vi "串口.vi"() -> ()   [LabVIEW 2012]
uses:
  <vilib>/Instr/_visa.llb/VISA Configure Serial Port (Instr).vi
  <vilib>/Utility/file.llb/Read From Spreadsheet File (I64).vi
  <vilib>/Utility/file.llb/Write To Spreadsheet File (I64).vi
panel:
  out "接收字节缓冲区":u8[](array[numeric])
  in  "选项卡控件":enum32{"帧采集", "采集信号", "信号回放"}(tab)
  out "时间：年月日-小时-分":string
  in  "保存数据格式":path=path "data.txt"
  out "卡车声":bool
  out "脚步声":bool
  in  "布尔 2":bool=TRUE
  in  "baud rate":u32=19200 caption="波特率"
  in  "VISA resource name":refnum<visa-resource-name>="COM1" caption="串口号"
  out "bytes read":u32=7 caption="读取的字节"
  in  "write":bool caption="写入"
  in  "string to write":string="*IDN?\n" caption="写入字符串"
  in  "read":bool=TRUE caption="读取"
  in  "data bits":u16=8 caption="数据比特" min=5 max=8 step=1
  in  "parity":u16(ring) caption="奇偶" items=["无", "奇", "偶", "标记", "空格"]
  in  "stop bits":u16(ring)=10 caption="停止位" items=["1.0"=10, "1.5"=15, "2.0"=20]
  in  "flow control":u16(ring) caption="流程控制" items=["无"=0, "XON/XOFF"=1, "RTS/CTS"=2, "DTR/DSR"=4]
  in  "delay before read (ms)":u32=1 caption="读取前延时(ms)"
  out "波形显示":cluster{u32, u32}(graph)
  out "read string":string="*IDN?\n" caption="读取字符串"
  in  "布尔":bool
  in  "保存帧格式":path=path "frame.txt"
  out "波形显示 2":u32[](graph) caption="波形显示"
  in  "数据位数":u16(ring)=8 items=["8"=8, "16"=16, "32"=32]
  in  "信号回放按键":bool
  out "波形显示 3":i64[][](graph) caption="波形显示"
  in  "数据格式文件":path=path "data.txt"
  # "1. 帧格式：\n    0xAA 类型 数据低字位 数据高字节 保留字节 保留字节 异或校验字节\n2. 类型： 0: nothing 1: 声方向 2: 目标类型 3: 过零率\n3. 此处无浏览按钮的路径都使用当前VI的相对路径"
  # "注：数据先低字节后高字节"
  # "1. 回放的信号文件必须是数据格式存储的文件\n2. 此处使用绝对路径"
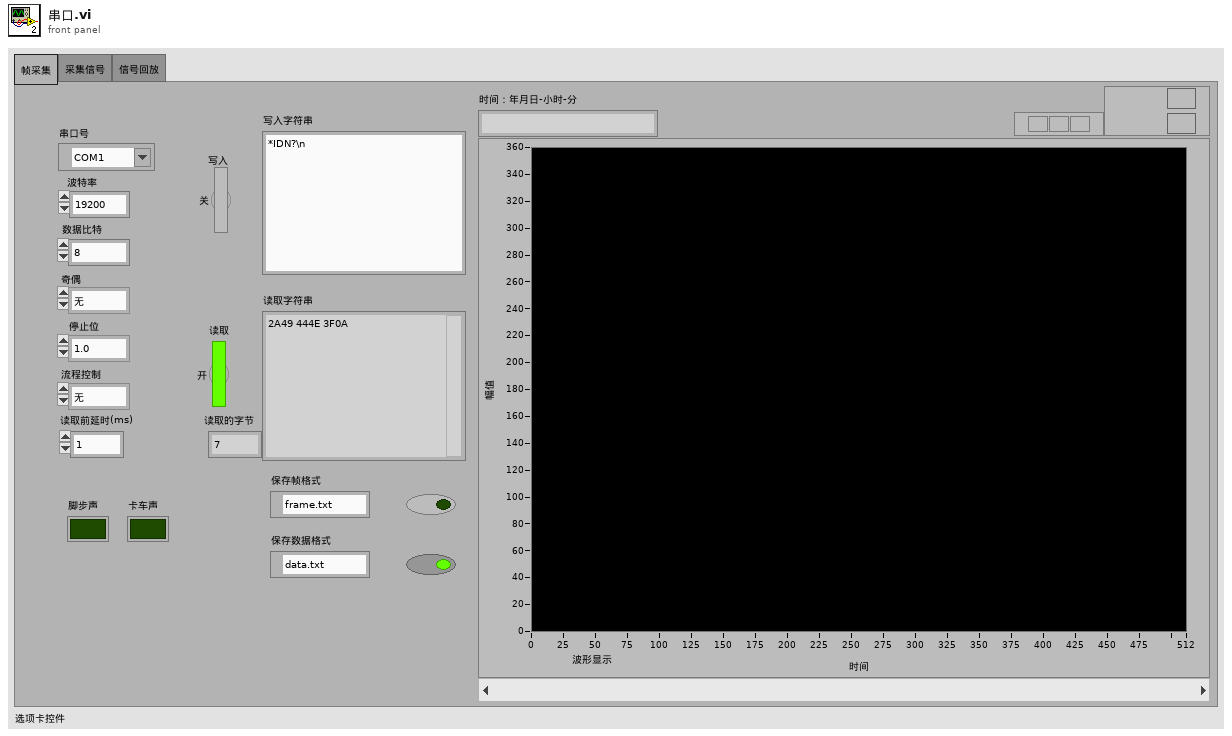
[diagram p1: front panel]
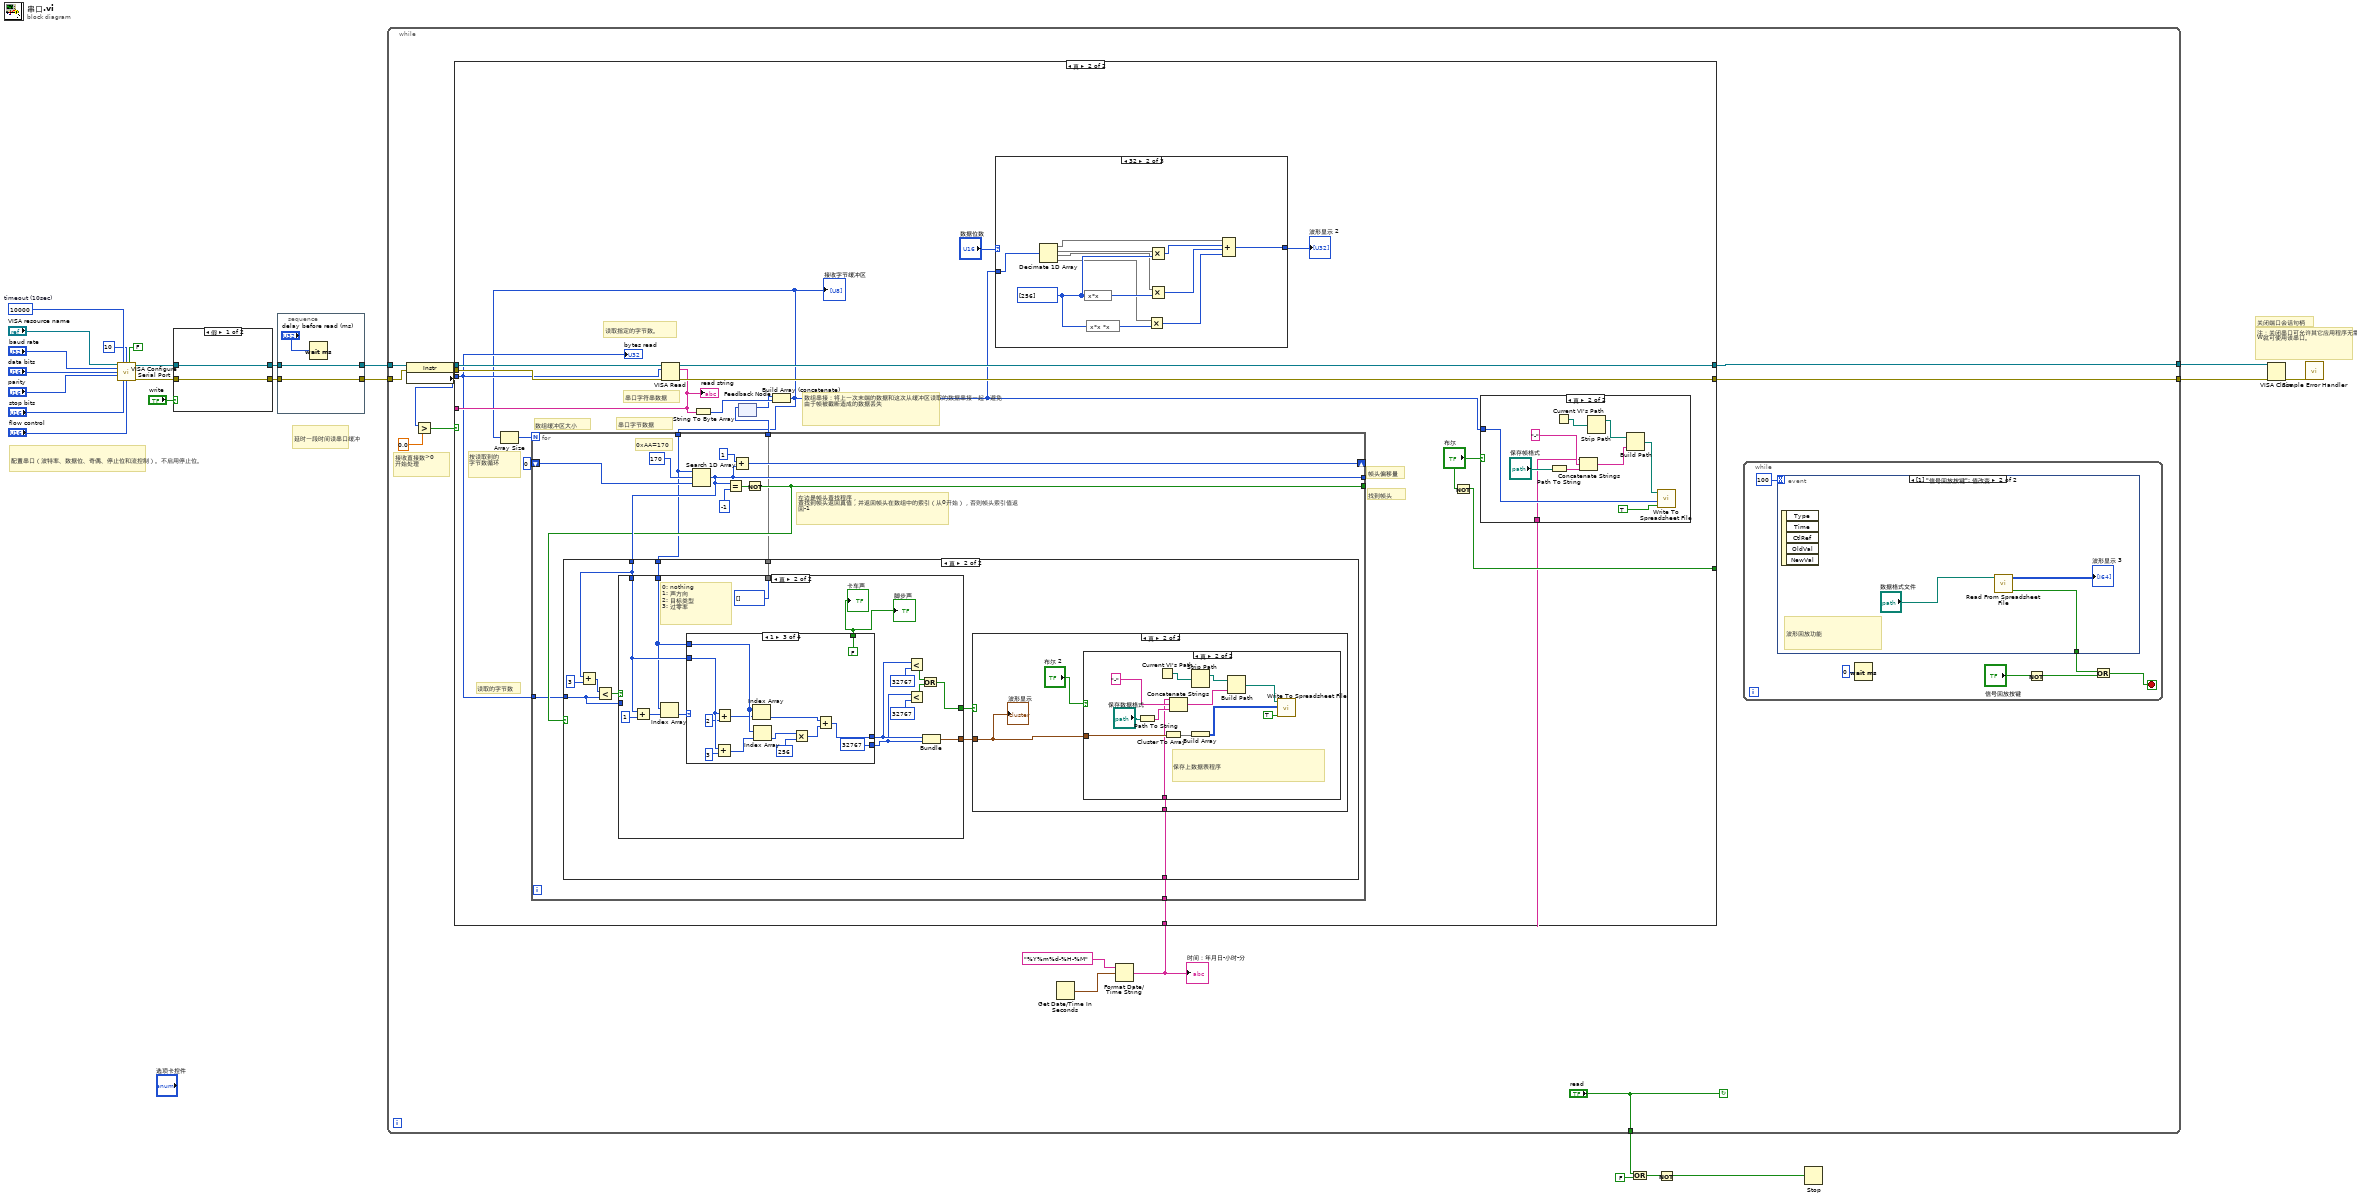
[diagram p0: block diagram]
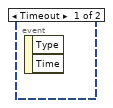
[diagram p2: hidden frame]
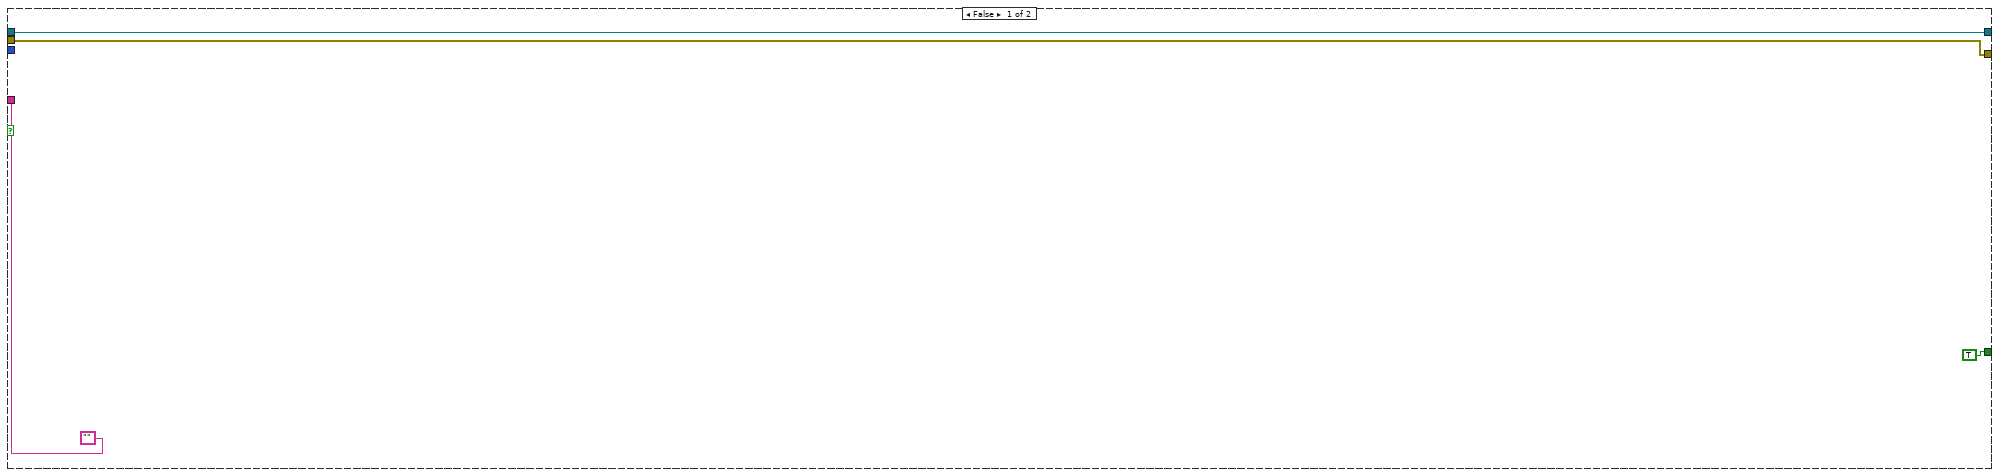
[diagram p3: hidden frame]
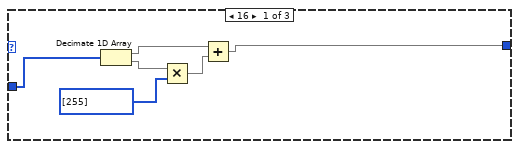
[diagram p4: hidden frame]
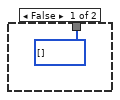
[diagram p7: hidden frame]
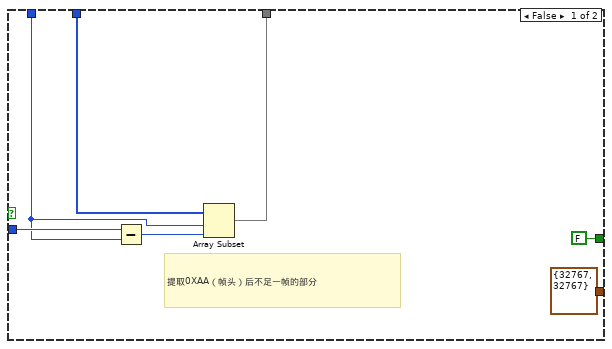
[diagram p8: hidden frame]
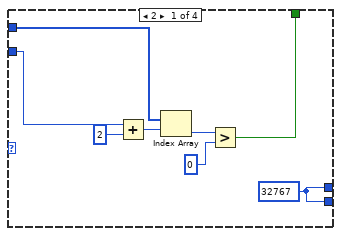
[diagram p9: hidden frame]
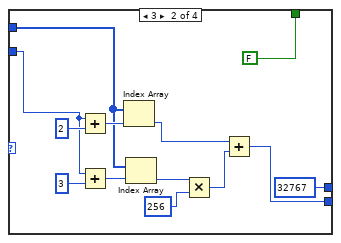
[diagram p10: hidden frame]
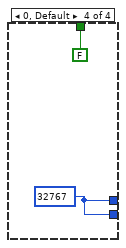
[diagram p11: hidden frame]
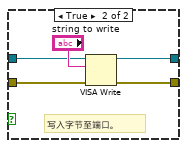
[diagram p14: hidden frame]
diagram:
  w15 = u32 10000  # timeout (10sec)
  # "延时一段时间读串口缓冲"
  # "注：关闭串口可允许其它应用程序无需退出LabVIEW就可使用该串口。"
  # "配置串口（波特率、数据位、奇偶、停止位和流控制）。不启用停止位。"
  # "关闭端口会话句柄"
  n1 = call-poly "VISA Configure Serial Port"("VISA resource name"="VISA resource name", "timeout (10sec)"=w15, "termination char\n(0xA = '\\n' = LF)"=u8 10 ("termination char\n(0xA = '\\n' = LF)"), "Enable Termination\nChar (T)"=FALSE ("Enable Termination\nChar (T)"), "baud rate (9600)"="baud rate", "data bits (8)"="data bits", "parity (0:none)"="parity", "stop bits (10: 1 bit)"="stop bits", "flow control (0:none)"="flow control") -> ("VISA resource name out"=w20:refnum<visa-resource-name>, "error out"=w21:errorcluster)  [unwired: 1 in, 4 out]
  n2 = case shown="假" "write" {
    tunnel: [w25 w30] -> w10
    tunnel: w20 -> [w24 w28]
    tunnel: w21 -> [w25 w27]
    tunnel: [w24 w26] -> w8
    frame False {
    }
    frame True {
      # "写入字节至端口。"
      n3 = VISA Write(VISA resource name=w28, write buffer="string to write", error in (no error)=w27) -> (VISA resource name out=w26:refnum<visa-resource-name>, error out=w30:errorcluster)  [unwired: 1 out]
    }
  }
  n4 = stacked-sequence {
    tunnel: w10 -> [w33]
    tunnel: [w33] -> w9
    tunnel: w8 -> [w32]
    tunnel: [w32] -> w7
    frame #0 {
      n5 = Wait (ms)(milliseconds to wait="delay before read (ms)") -> ()  [unwired: 1 out]
    }
  }
  n6 = while {
    tunnel: [w46] -> w19
    tunnel: [w45] -> w18
    tunnel: w9 -> [w44]
    tunnel: w7 -> [w43]
    tunnel: ["read"] -> w5
    stop <- "read" continue-if-true
    # "接收直接数>0\n开始处理"
    n7 = property class="Instr"(reference=w43, error in=w44) -> (reference out=w42:refnum<visa-resource-name>, error out=w41:errorcluster, "Serial Settings:Number of Bytes at Serial Port"=w39:u32)
    n8 = Greater?(x=w39, y=0.0) -> (0:w37:bool)
    n9 = Get Date/Time In Seconds() -> (seconds since 1Jan1904=w36:timestamp)
    n10 = Format Date/Time String(time format string (%c)="%Y%m%d-%H-%M" ("时间格式字符串(%c)"), seconds (now)=w36) -> (date/time string=w34:string)  [unwired: 1 in]
    "时间：年月日-小时-分" <- w34
    n11 = case shown="真" w37 {
      tunnel: [w57 w76] -> w46
      tunnel: [w58 w73] -> w45
      tunnel: w42 -> [w58 w75]
      tunnel: w41 -> [w57 w74]
      tunnel: w39 -> [_ w67]
      tunnel: ["" w71] -> _
      tunnel: [TRUE w69] -> _
      tunnel: w34 -> [_ w68]
      frame False {
      }
      frame True {
        # "串口字符串数据"
        # "串口字节数据"
        # "按读取到的\n字节数循环"
        # "数组串接：将上一次末端的数据和这次从缓冲区读取的数据串接一起，避免由于帧被截断造成的数据丢失"
        # "读取的字节数"
        # "数组缓冲区大小"
        # "找到帧头"
        # "帧头偏移量"
        # "读取指定的字节数。"
        n12 = VISA Read(VISA resource name=w75, byte count=w67, error in (no error)=w74) -> (VISA resource name out=w73:refnum<visa-resource-name>, read buffer=w71:string, error out=w76:errorcluster)  [unwired: 1 out]
        "read string" <- w71
        n13 = String To Byte Array ("字符串转字节函数")(string=w71) -> (unsigned byte array=w65:u8[])
        n14 = feedback #1() -> (w64:u8[])  [unwired: 1 in]
        n15 = Build Array (concatenate)(w64, w65) -> (w60:u8[])
        "接收字节缓冲区" <- w60
        n16 = Array Size(array=w60) -> (size(s)=w63:i32)
        n17 = for {
          N: w63 -> [_]
          shift-right: [w114] -> _
          shift-left: 0 -> [w116]
          tunnel: [w111] -> _
          tunnel: [w110] -> _
          tunnel: w60 -> [w109]
          tunnel: w68 -> [w108]
          tunnel: w67 -> [w107]
          tunnel: [w106] -> w66
          # "左边是帧头查找程序，\n查找到帧头返回真值，并返回帧头在数组中的索引（从0开始），否则帧头索引值返回-1"
          # "0xAA=170"
          n18 = Search 1D Array(1D array=w109, element=u8 170 ("元素"), start index (0)=w116) -> (index of element=w111:i32)
          n19 = Equal?(x=w111, y=-1) -> (x = y?=w112:bool)
          n20 = Add(x=1, y=w111) -> (x+y=w114:i32)
          n21 = Not(x=w112) -> (.not. x?=w110:bool)
          n22 = case shown="真" w110 {
            tunnel: w111 -> [_ w120]
            tunnel: w109 -> [_ w128]
            tunnel: w108 -> [_ w125]
            tunnel: w107 -> [_ w121]
            tunnel: [u8[] [] w119] -> w106
            frame False {
            }
            frame True {
              n23 = Add(x=w120, y=u32 3) -> (x+y=w122:u32)
              n24 = Less?(x=w122, y=w121) -> (x < y?=w123:bool)
              n25 = case shown="真" w123 {
                tunnel: w120 -> [w131 w148]
                tunnel: w128 -> [w130 w147]
                tunnel: [cluster{u32, u32} {32767, 32767} w143] -> w127
                tunnel: [FALSE w137] -> w126
                tunnel: w121 -> [w133 _]
                tunnel: [w129 u8[] []] -> w119
                frame False {
                  # "提取0XAA（帧头）后不足一帧的部分"
                  n26 = Subtract(x=w133, y=w131) -> (x-y=w132:u32)
                  n27 = Array Subset(array=w130, index=w131, length=w132) -> (w129:u8[])
                }
                frame True {
                  # "0: nothing\n1: 声方向\n2: 目标类型\n3: 过零率"
                  n28 = Add(x=w148, y=u8 1) -> (x+y=w149:i32)
                  n29 = Index Array(array=w147, index=w149) -> (element=w146:u8)
                  n30 = case shown="1" w146 {
                    tunnel: w148 -> [w158 w169 w184 _]
                    tunnel: w147 -> [w155 w166 w183 _]
                    tunnel: [w152 FALSE FALSE FALSE] -> w145
                    tunnel: [w151 u32 32767 w173 w185] -> w141
                    tunnel: [w151 w160 u32 32767 w185] -> w140
                    frame 2 {
                      w151 = u32 32767
                      n31 = Add(x=w158, y=2) -> (x+y=w156:i32)
                      n32 = Index Array(array=w155, index=w156) -> (element=w154:u8)
                      n33 = Greater?(x=w154, y=u8 0) -> (0:w152:bool)
                    }
                    frame 3 {
                      n34 = Add(x=w169, y=2) -> (x+y=w170:i32)
                      n35 = Add(x=w169, y=3) -> (x+y=w167:i32)
                      n36 = Index Array(array=w166, index=w170) -> (element=w162:u8)
                      n37 = Index Array(array=w166, index=w167) -> (element=w165:u8)
                      n38 = Multiply(x=w165, y=u32 256) -> (x*y=w163:u32)
                      n39 = Add(x=w162, y=w163) -> (x+y=w160:u32)
                    }
                    frame 1 {
                      n40 = Add(x=w184, y=3 ("索引")) -> (x+y=w177:i32)
                      n41 = Add(x=w184, y=2 ("索引")) -> (x+y=w180:i32)
                      n42 = Index Array(array=w183, index=w180) -> (element=w182:u8)
                      n43 = Index Array(array=w183, index=w177) -> (element=w176:u8)
                      n44 = Multiply(x=w176, y=u32 256 ("x")) -> (x*y=w181:u32)
                      n45 = Add(x=w182, y=w181) -> (x+y=w173:u32)
                    }
                    frame 0, Default {
                      w185 = u32 32767
                    }
                  }
                  "卡车声" <- w145
                  "脚步声" <- w145
                  n46 = Less?(x=w141, y=u32 32767) -> (x < y?=w138:bool)
                  n47 = Less?(x=w140, y=u32 32767) -> (x < y?=w139:bool)
                  n48 = Or(x=w138, y=w139) -> (x .or. y?=w137:bool)
                  n49 = Bundle(w141, w140) -> (w143:cluster{u32, u32})  [unwired: 1 in]
                }
              }
              n50 = case shown="真" w126 {
                tunnel: w127 -> [_ w187]
                tunnel: w125 -> [_ w188]
                frame False {
                }
                frame True {
                  n51 = case shown="真" "布尔 2" {
                    tunnel: w187 -> [_ w200]
                    tunnel: w188 -> [_ w191]
                    frame False {
                    }
                    frame True {
                      # "保存上数据表程序"
                      n52 = Path To String(path="保存数据格式") -> (string=w193:string)
                      n53 = Current VI's Path() -> (path=w197:path)
                      n54 = Cluster To Array(cluster=w200) -> (array=w199:u32[])
                      n55 = Concatenate Strings(w191, "-" ("字符串"), w193) -> (w190:string)
                      n56 = Strip Path(path=w197) -> (stripped path=w196:path)  [unwired: 1 out]
                      n57 = Build Array(w199) -> (w198:u32[][])
                      n58 = Build Path(base path=w196, name or relative path=w190) -> (appended path=w195:path)
                      n59 = call-poly <vilib>:"Write To Spreadsheet File.vi"("append to file? (new file:F)"=TRUE, "2D data"=w198, "file path (dialog if empty)"=w195) -> ()  [unwired: 5 in, 1 out]
                    }
                  }
                  "波形显示" <- w187
                }
              }
            }
          }
        }
        n60 = feedback-in #1(w66) -> ()
        n61 = case shown="32" "数据位数" {
          tunnel: [w77 w83 w95] -> w61
          tunnel: w60 -> [w82 w94 w95]
          frame 16 {
            n62 = Decimate 1D Array(w82) -> (w78:u8[], w81:u8[])
            n63 = Multiply(x=w81, y=u8[] [255]) -> (x*y=w79:u8[])
            n64 = Add(x=w78, y=w79) -> (x+y=w77:u8[])
          }
          frame 32 {
            w90 = u32[] [256] ("y")
            n65 = Decimate 1D Array(w94) -> (w87:u8[], w93:u8[], w89:u8[], w88:u8[])
            n66 = expression code="x*x"(w90) -> (w92:u32[])
            n67 = expression code="x*x *x"(w90) -> (w91:u32[])
            n68 = Multiply(x=w88, y=w91) -> (x*y=w84:u32[])
            n69 = Multiply(x=w93, y=w90) -> (x*y=w86:u32[])
            n70 = Multiply(x=w89, y=w92) -> (x*y=w85:u32[])
            n71 = Compound Arithmetic op=ADD(w87, w86, w85, w84) -> (w83:u32[])
          }
          frame 8, Default {
          }
        }
        "波形显示 2" <- w61
        n72 = Not(x="布尔") -> (.not. x?=w69:bool)
        n73 = case shown="真" "布尔" {
          tunnel: w60 -> [_ w105]
          tunnel: w68 -> [_ w97]
          frame False {
          }
          frame True {
            n74 = Path To String(path="保存帧格式") -> (string=w99:string)
            n75 = Current VI's Path() -> (path=w103:path)
            n76 = Concatenate Strings(w97, "-" ("字符串"), w99) -> (w96:string)
            n77 = Strip Path(path=w103) -> (stripped path=w102:path)  [unwired: 1 out]
            n78 = Build Path(base path=w102, name or relative path=w96) -> (appended path=w101:path)
            n79 = call-poly <vilib>:"Write To Spreadsheet File.vi"("append to file? (new file:F)"=TRUE, "1D data"=w105, "file path (dialog if empty)"=w101) -> ()  [unwired: 5 in, 1 out]
          }
        }
        "bytes read" <- w67
      }
    }
    n80 = while {
      stop <- w47 stop-if-true
      n81 = event shown="[1] \"信号回放按键\": 值改变" {
        selector: _ -> [_ _]
        dyn-events: _ -> [_ _]
        timeout: 100 -> [_ _]
        tunnel: [_ w54] -> w49
        event Timeout {
          n82 = event-data() -> ()  [unwired: 1 in, 2 out]
        }
        event "信号回放按键": Value Change {
          # "波形回放功能"
          n83 = event-data() -> ()  [unwired: 1 in, 5 out]
          n84 = call-poly <vilib>:"Read From Spreadsheet File.vi"("file path (dialog if empty)"="数据格式文件") -> ("EOF?"=w54:bool, "all rows"=→"波形显示 3":i64[][])  [unwired: 6 in, 3 out]
        }
      }
      n85 = Wait (ms)(milliseconds to wait=u32 0 ("等待时间（毫秒）")) -> ()  [unwired: 1 out]
      n86 = Not(x="信号回放按键") -> (.not. x?=w48:bool)
      n87 = Or(x=w49, y=w48) -> (x .or. y?=w47:bool)
    }
  }
  n88 = Or(x=w5, y=FALSE) -> (x .or. y?=w6:bool)
  n89 = Not(x=w6) -> (.not. x?=w3:bool)
  n90 = Stop(stop? (T)=w3) -> ()
  n91 = VISA Close(VISA resource name=w18, error in (no error)=w19) -> (error out=w17:errorcluster)
  n92 = call <vilib>:"Simple Error Handler.vi"("error in (no error)"=w17) -> ()  [unwired: 1 in, 8 out]
